vi "Close.vi"(8 "Error In":errorcluster, 11 "Process In":refnum<class "Process.lvclass">) -> (0 "Error Out":errorcluster)   [LabVIEW 2019, in "Process.lvclass"]
uses:
  Process.lvclass
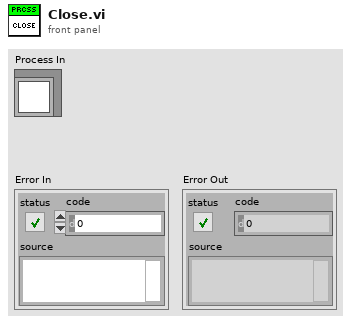
[diagram p1: front panel]
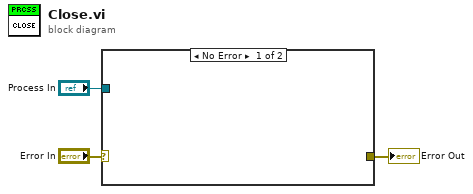
[diagram p0: block diagram]
diagram:
  n1 = case shown="No Error" "Error In" {
    selector: "Error In" -> [_ w4]
    tunnel: [_ w4] -> w2
    tunnel: "Process In" -> [_ _]
    frame No Error {
    }
    frame Error {
    }
  }
  "Error Out" <- w2
